vi "AddDiffPulseVoltammetry.vi"(0 "deviceName":string, 1 "channel":u8, 2 "repeats":u16=1, 3 "quietTime":sgl, 4 "quietTimeSamplingInterval":sgl, 5 "startVoltage":sgl, 6 "isStartVoltageVsOCP":bool, 7 "error in (no error)":errorcluster, 8 "endVoltage":sgl, 9 "isEndVoltageVsOCP":bool, 10 "vStep":sgl, 11 "pulseHeight":sgl, 12 "pulseWidth":sgl, 13 "pulsePeriod":sgl, 14 "approxMaxCurrent":sgl=inf, 15 "isAutoRange":bool=TRUE, 16 "alphaFactor":sgl=75.0) -> (27 "error out":errorcluster)   [LabVIEW 2018]
doc: "EXPORT void AisAddDiffPulseVoltammetry(const char* deviceName, uint8_t channel, uint16_t repeats, float quietTime, float quietTimeSamplingInterval, float startVoltage, bool isStartVoltageVsOCP, float endVoltage, bool isEndVoltageVsOCP, float vStep, float pulseHeight, float pulseWidth, float pulsePeriod, float approxMaxCurrent, bool isAutoRange, float alphaFactor);"
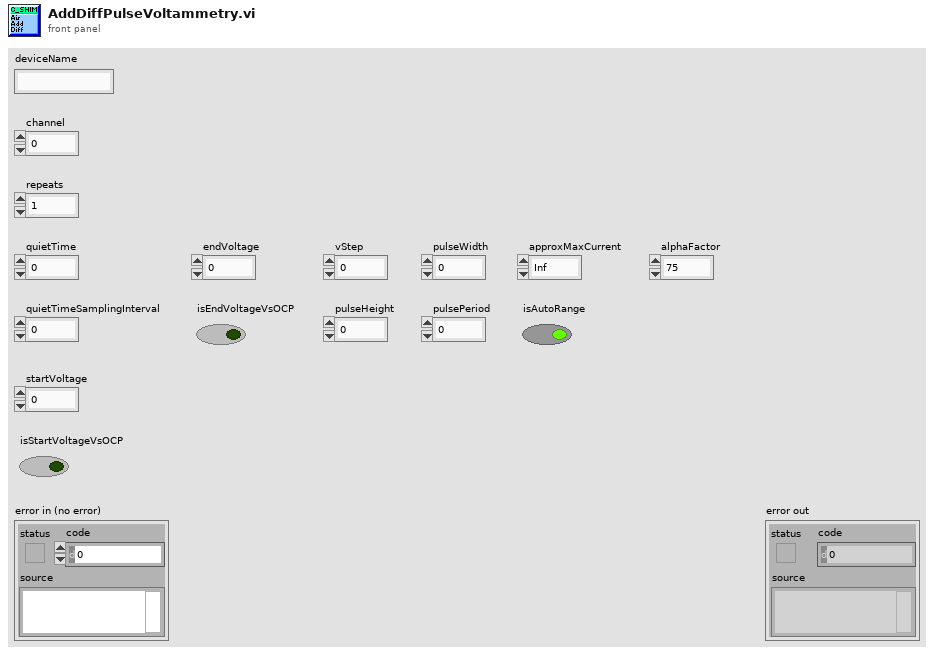
[diagram p1: front panel]
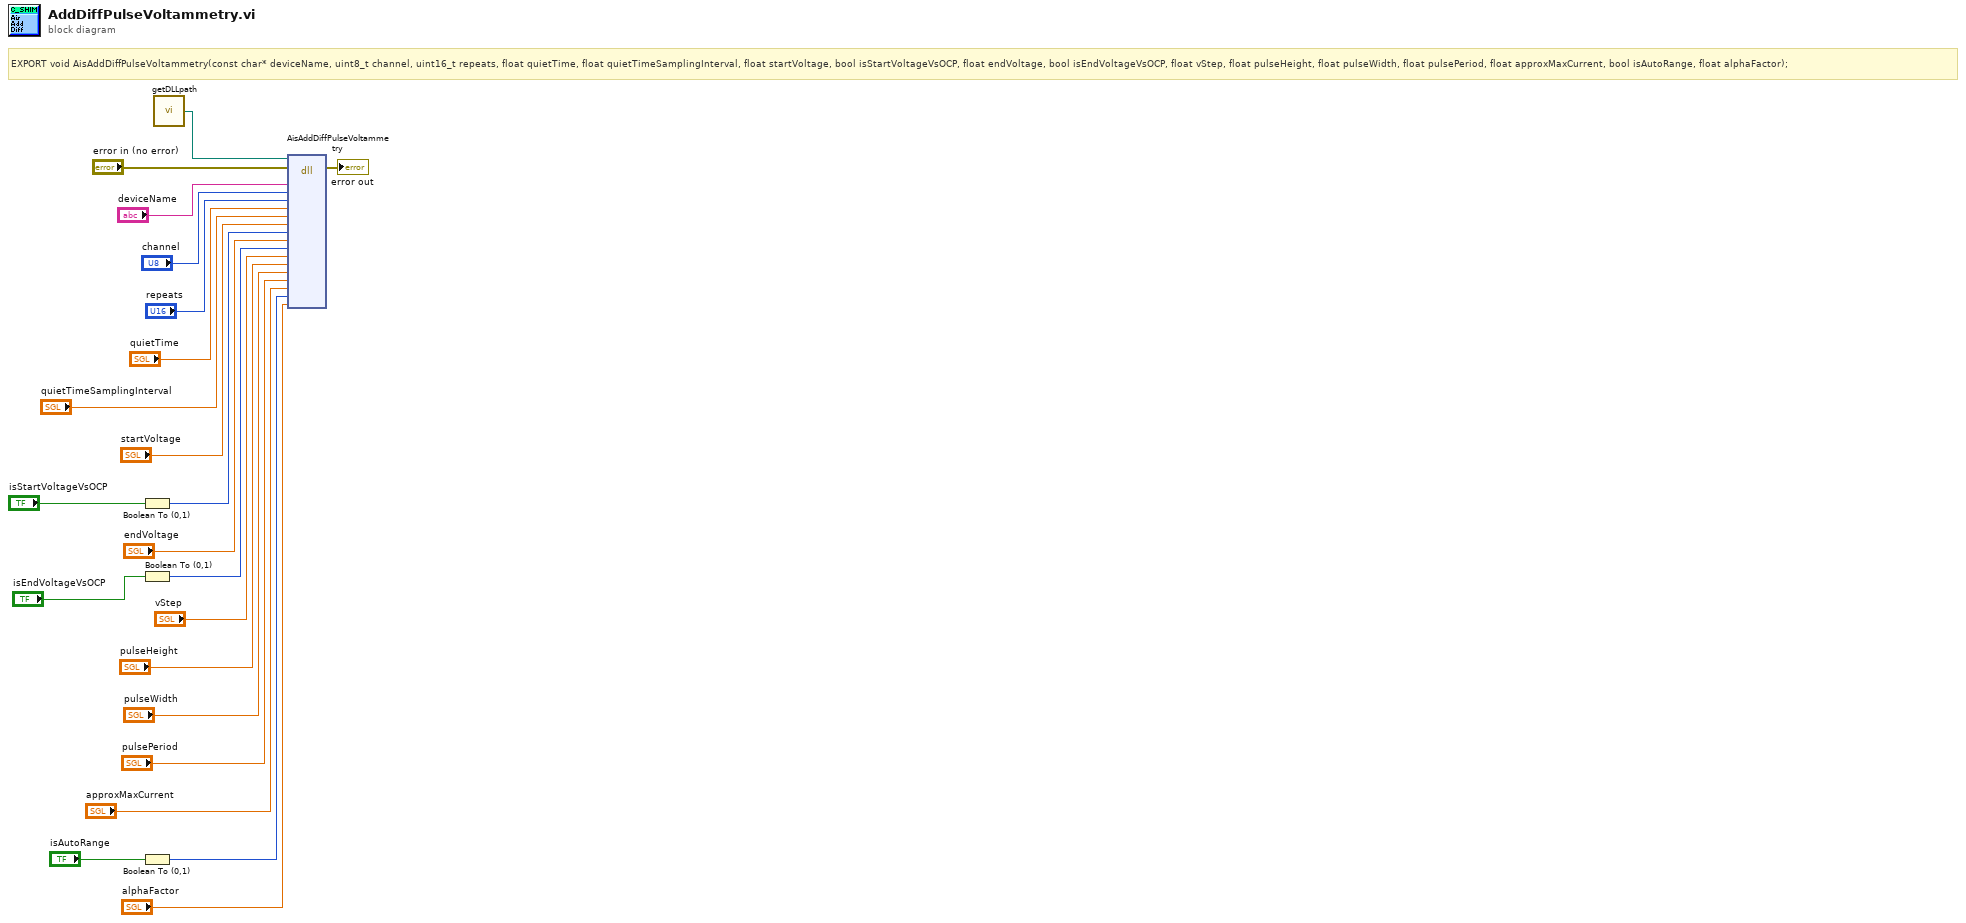
[diagram p0: block diagram]
diagram:
  # "EXPORT void AisAddDiffPulseVoltammetry(const char* deviceName, uint8_t channel, uint16_t repeats, float quietTime, float quietTimeSamplingInterval, float startVoltage, bool isStartVoltageVsOCP, float endVoltage, bool isEndVoltageVsOCP, float vStep, float pulseHeight, float pulseWidth, float pulsePeriod, float approxMaxCurrent, bool isAutoRange, float alphaFactor);"
  n1 = Boolean To (0,1)(Boolean="isStartVoltageVsOCP") -> (0, 1=w15:i16)
  n2 = Boolean To (0,1)(Boolean="isEndVoltageVsOCP") -> (0, 1=w12:i16)
  n3 = Boolean To (0,1)(Boolean="isAutoRange") -> (0, 1=w5:i16)
  n4 = call "getDLLpath.vi"() -> ("DLL_Path"=w1:path)
  n5 = dll-call lib="?" fn="AisAddDiffPulseVoltammetry"(path in=w1, error in="error in (no error)", "deviceName"="deviceName", "channel"="channel", "repeats"="repeats", "quietTime"="quietTime", "quietTimeSamplingInterval"="quietTimeSamplingInterval", "startVoltage"="startVoltage", "isStartVoltageVsOCP"=w15, "endVoltage"="endVoltage", "isEndVoltageVsOCP"=w12, "vStep"="vStep", "pulseHeight"="pulseHeight", "pulseWidth"="pulseWidth", "pulsePeriod"="pulsePeriod", "approxMaxCurrent"="approxMaxCurrent", "isAutoRange"=w5, "alphaFactor"="alphaFactor") -> (error out=→"error out":errorcluster)  [unwired: 18 in, 1 out]
